vi "Notifiers - Get.vi"(8 "error in":errorcluster) -> (0 "error out":errorcluster, 3 "ECU Notifiers":T1)   [LabVIEW 2024, in "ECU InterComm.lvlib"]
uses:
  ECU InterComm.lvlib
  ECU Notifiers.ctl
  General Actions.ctl
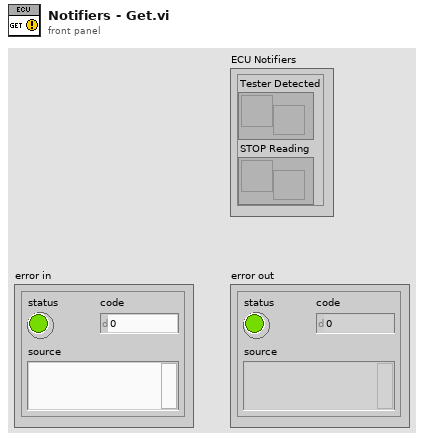
[diagram p1: front panel]
types:
  T1 = typedef "ECU InterComm.lvlib/ECU Notifiers.ctl" = cluster{"Tester Detected":refnum<notifier>, "STOP Reading":refnum<notifier>}
  T2 = typedef "ECU InterComm.lvlib/General Actions.ctl" = enum16{"Create", "Get", "Destroy"}
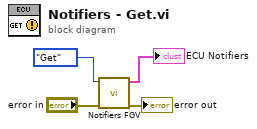
[diagram p0: block diagram]
diagram:
  n1 = call "Notifiers FGV.vi"("error in"="error in", "Notifier Action"=General_Actions."Get") -> ("error out"=→"error out":errorcluster, "ECU Notifiers"=→"ECU Notifiers":T1)  [unwired: 8 in]
